vi "Turn Supply On or Off.vi"(0 "Supply Handle in":refnum<k15>, 1 "Channel Name(s)":string, 5 "Power On":bool, 11 "error in (no error)":errorcluster) -> (4 "Supply Handle out":refnum<k15>, 15 "error out":errorcluster)   [LabVIEW 2016, in "Supply.lvlib"]
uses:
  Supply.lvlib
  <instrlib>/niDCPower/nidcpower.llb/niDCPower Wait For Event - Event.ctl
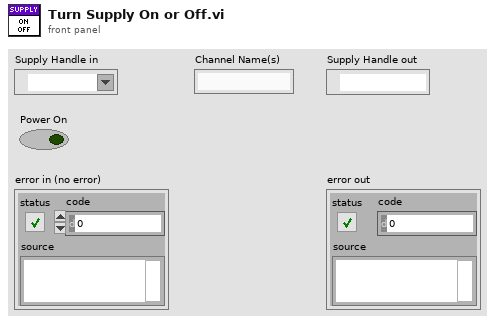
[diagram p1: front panel]
types:
  T1 = typedef "niDCPower Wait For Event - Event.ctl" = i32
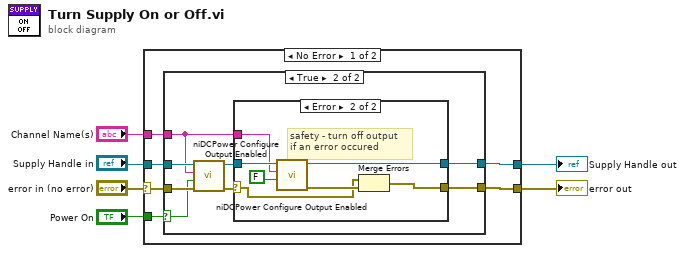
[diagram p0: block diagram]
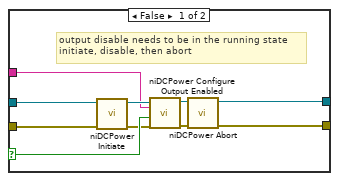
[diagram p2: hidden frame]
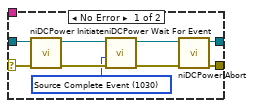
[diagram p3: hidden frame]
diagram:
  n1 = case shown="No Error" "error in (no error)" {
    selector: "error in (no error)" -> [w12 w48]
    tunnel: "Supply Handle in" -> [w11 w47]
    tunnel: "Power On" -> [w10 _]
    tunnel: [w9 w48] -> w3
    tunnel: [w8 w47] -> w2
    tunnel: "Channel Name(s)" -> [w7 _]
    frame No Error {
      n2 = case shown="True" w10 {
        selector: w10 -> [w21 w24]
        tunnel: w12 -> [w22 w30]
        tunnel: w11 -> [w18 w26]
        tunnel: [w16 w29] -> w9
        tunnel: [w14 w28] -> w8
        tunnel: w7 -> [w13 w23]
        frame False {
          # "output disable needs to be in the running state\ninitiate, disable, then abort"
          n3 = call <instrlib>:"niDCPower Initiate.vi"("error in (no error)"=w22, "instrument handle"=w18) -> ("error out"=w19:errorcluster, "instrument handle out"=w17:refnum<k15>)  [unwired: 8 in]
          n4 = call <instrlib>:"niDCPower Configure Output Enabled.vi"("error in (no error)"=w19, "output enabled"=w21, "channel name"=w13, "instrument handle"=w17) -> ("error out"=w20:errorcluster, "instrument handle out"=w15:refnum<k15>)  [unwired: 6 in]
          n5 = call <instrlib>:"niDCPower Abort.vi"("error in (no error)"=w20, "instrument handle"=w15) -> ("error out"=w16:errorcluster, "instrument handle out"=w14:refnum<k15>)  [unwired: 8 in]
        }
        frame True {
          n6 = call <instrlib>:"niDCPower Configure Output Enabled.vi"("error in (no error)"=w30, "output enabled"=w24, "channel name"=w23, "instrument handle"=w26) -> ("error out"=w27:errorcluster, "instrument handle out"=w25:refnum<k15>)  [unwired: 6 in]
          n7 = case shown="Error" w27 {
            selector: w27 -> [w34 w41]
            tunnel: w25 -> [w33 w46]
            tunnel: [w32 w42] -> w29
            tunnel: [w31 w44] -> w28
            tunnel: w23 -> [_ w40]
            frame No Error {
              w35 = T1 1030 items=["Source Complete Event"=1030, "Measure Complete Event"=1031, "Sequence Iteration Complete Event"=1032, "Sequence Engine Done Event"=1033, "Pulse Complete Event"=1051, "Ready For Pulse Trigger Event"=1052] ("event")
              n8 = call <instrlib>:"niDCPower Initiate.vi"("error in (no error)"=w34, "instrument handle"=w33) -> ("error out"=w36:errorcluster, "instrument handle out"=w37:refnum<k15>)  [unwired: 8 in]
              n9 = call <instrlib>:"niDCPower Wait For Event.vi"("error in (no error)"=w36, "event"=w35, "instrument handle"=w37) -> ("error out"=w39:errorcluster, "instrument handle out"=w38:refnum<k15>)  [unwired: 7 in]
              n10 = call <instrlib>:"niDCPower Abort.vi"("error in (no error)"=w39, "instrument handle"=w38) -> ("error out"=w32:errorcluster, "instrument handle out"=w31:refnum<k15>)  [unwired: 8 in]
            }
            frame Error {
              # "safety - turn off output\nif an error occured"
              n11 = call <instrlib>:"niDCPower Configure Output Enabled.vi"("output enabled"=FALSE, "channel name"=w40, "instrument handle"=w46) -> ("error out"=w43:errorcluster, "instrument handle out"=w44:refnum<k15>)  [unwired: 7 in]
              n12 = Merge Errors(w41, w43) -> (w42:errorcluster)
            }
          }
        }
      }
    }
    frame Error {
    }
  }
  "error out" <- w3
  "Supply Handle out" <- w2
